vi "Lift E Stop.vi"   [LabVIEW 2014]
uses:
  Global Variables.vi
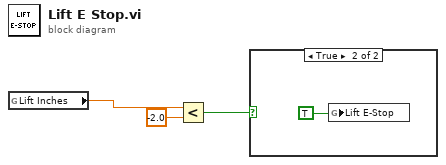
[diagram p0: block diagram]
diagram:
  n1 = global read "Global Variables.vi" "Lift Inches"() -> (w3:dbl)
  n2 = Less?(x=w3, y=-2.0) -> (x < y?=w1:bool)
  n3 = case shown="True" w1 {
    frame False {
    }
    frame True {
      n4 = global write "Global Variables.vi" "Lift E-Stop"(TRUE) -> ()
    }
  }
